vi "CSM - Global Log Event.vi"(6 "timeout in ms (5000ms)":i32=5000, 8 "Error in":errorcluster caption="Error in (no error)") -> (0 "Error out":errorcluster, 3 "CSM Global Log Event":refnum<user-event>)   [LabVIEW 2020, in "Communicable State Machine.lvlib"]
doc: "Obtain CSM Global Log Event Reference.\n\n<b>Inputs:</b>\n - <b>Error in</b>: Error cluster\n\n<b>Outputs:</b>\n - <b>CSM Global Log Event</b>: User event reference for CSM global log.\n - <b>Error out</b>: Error cluster"
uses:
  Communicable State Machine.lvlib
  _CSM_GlobalLog_MSG.ctl
  _CSM_Response Source Message.ctl
  _CSM_GlobalLog_MSG_TYPE.ctl
  GEvt-RequestDef.ctl
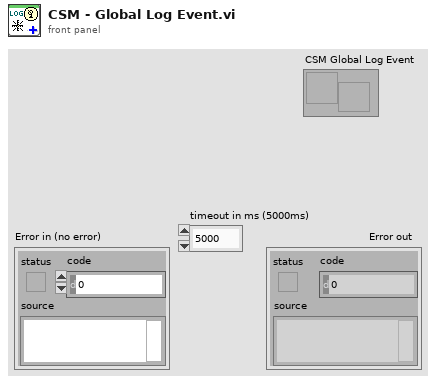
[diagram p1: front panel]
types:
  T1 = typedef "Communicable State Machine.lvlib/GEvt-RequestDef.ctl" = cluster{"Operation":enum16{"Obtain", "Destroy", "Force Destroy"}, "RespQ":refnum<queue>, "CSM Global Log Event":refnum<user-event>}
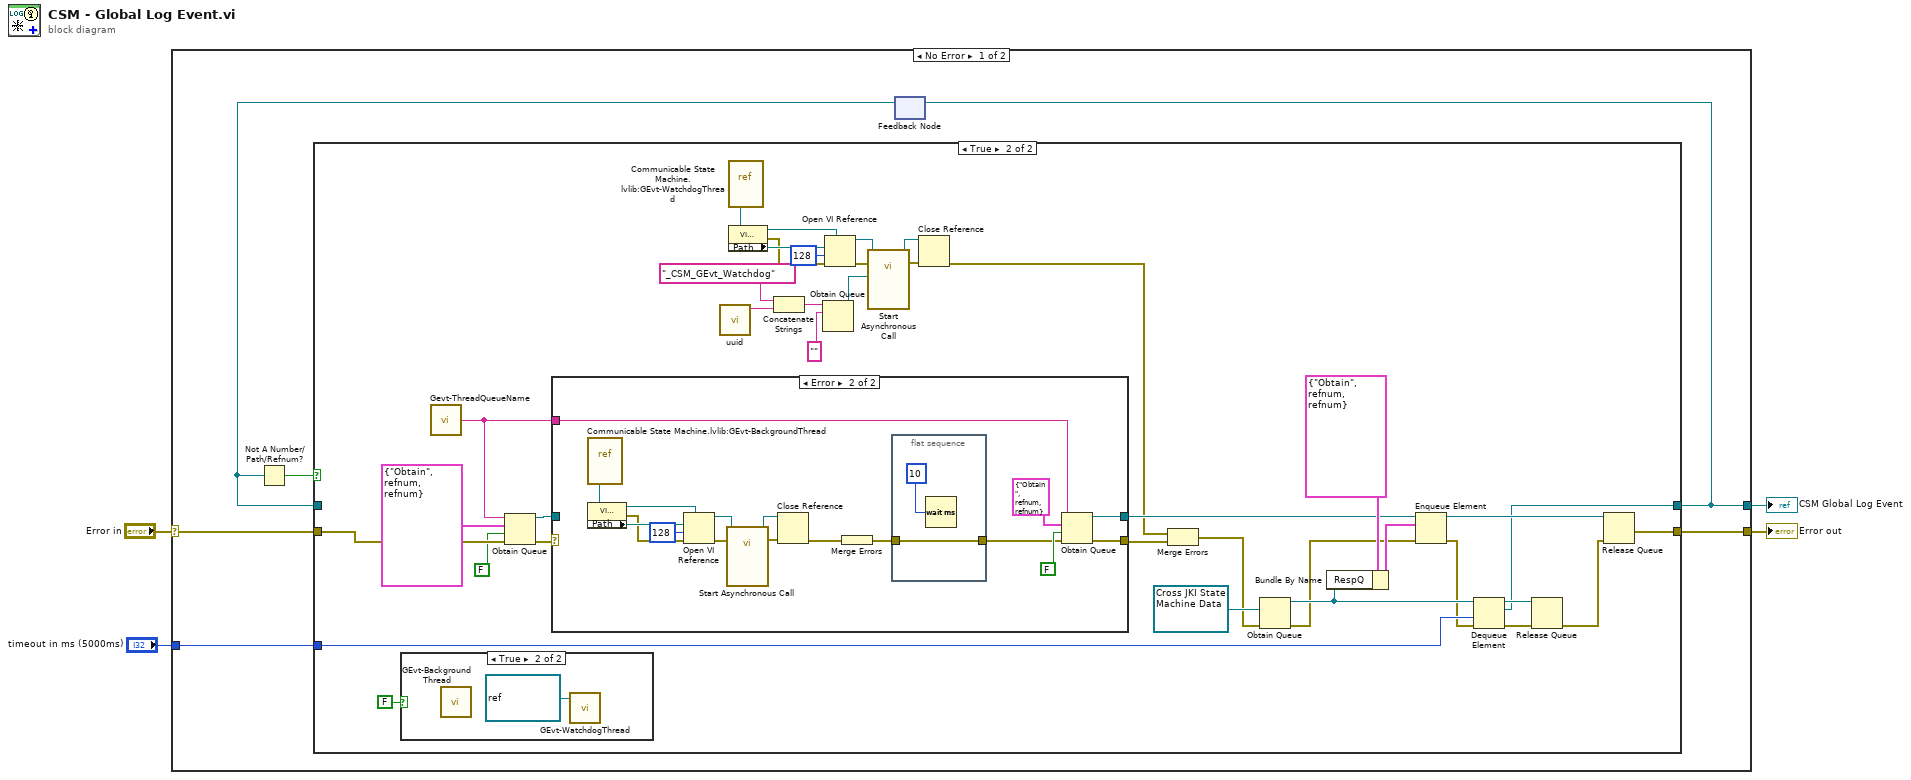
[diagram p0: block diagram]
diagram:
  n1 = case shown="No Error" "Error in" {
    selector: "Error in" -> [w8 w73]
    tunnel: [w10 w73] -> w4
    tunnel: [w7 _] -> w2
    tunnel: "timeout in ms (5000ms)" -> [w9 _]
    frame No Error {
      n2 = feedback #1() -> (w5:refnum<user-event>)  [unwired: 1 in]
      n3 = Not A Number/Path/Refnum?(number/path/refnum=w5) -> (NaN/Path/Refnum?=w6:bool)
      n4 = case shown="True" w6 {
        tunnel: [w11 w50] -> w10
        tunnel: w9 -> [_ w49]
        tunnel: w8 -> [w11 w48]
        tunnel: [w12 w29] -> w7
        tunnel: w5 -> [w12 _]
        frame False {
        }
        frame True {
          n5 = case shown="True" FALSE {
            frame False {
            }
            frame True {
              n6 = call "GEvt-BackgroundThread.vi"() -> ()  [unwired: 12 in]
              n7 = call "GEvt-WatchdogThread.vi"("WatchDogQ"=refnum<queue> refnum) -> ()  [unwired: 11 in]
            }
          }
          n8 = call "Gevt-ThreadQueueName.vi"() -> ("ThreadQueueName"=w31:string)  [unwired: 5 in]
          n9 = Obtain Queue(name (unnamed)=w31, element data type=T1 {"Operation"=enum."Obtain", "RespQ"=refnum, "CSM Global Log Event"=refnum}, create if not found? (T)=FALSE, error in (no error)=w48) -> (queue out=w44:refnum<queue>, error out=w45:errorcluster)  [unwired: 1 in, 1 out]
          n10 = case shown="Error" w45 {
            selector: w45 -> [w53 _]
            tunnel: w44 -> [w52 _]
            tunnel: [w53 w57] -> w38
            tunnel: [w52 w56] -> w39
            tunnel: w31 -> [_ w55]
            frame No Error {
            }
            frame Error {
              n11 = vi-ref "Communicable State Machine.lvlib:GEvt-BackgroundThread.vi"() -> (w69:refnum<vi>)
              n12 = property class="VI (strict)"(reference=w69) -> (reference out=w65:refnum<vi>, error out=w67:errorcluster, "Path"=w68:path)  [unwired: 1 in]
              n13 = Open VI Reference(type specifier VI Refnum (for type only)=w65, vi path=w68, options=128, error in (no error)=w67) -> (vi reference=w66:refnum<vi>, error out=w70:errorcluster)  [unwired: 2 in]
              n14 = call-by-ref "Start Asynchronous Call"(reference=w66, error in=w70) -> (reference out=w63:refnum<vi>, error out=w64:errorcluster)  [unwired: 12 in]
              n15 = Close Reference(reference=w63, error in (no error)=w64) -> (error out=w61:errorcluster)
              n16 = Merge Errors(w61) -> (w54:errorcluster)
              n17 = flat-sequence {
                tunnel: [w71] -> w58
                tunnel: w54 -> [w71]
                frame #0 {
                  n18 = Wait (ms)(milliseconds to wait=u32 10) -> ()  [unwired: 1 out]
                }
              }
              n19 = Obtain Queue(name (unnamed)=w55, element data type=T1 {"Operation"=enum."Obtain", "RespQ"=refnum, "CSM Global Log Event"=refnum}, create if not found? (T)=FALSE, error in (no error)=w58) -> (queue out=w56:refnum<queue>, error out=w57:errorcluster)  [unwired: 1 in, 1 out]
            }
          }
          n20 = call "uuid.vi"() -> ("UUID"=w24:string)  [unwired: 11 in]
          n21 = vi-ref "Communicable State Machine.lvlib:GEvt-WatchdogThread.vi"() -> (w22:refnum<vi>)
          n22 = property class="VI (strict)"(reference=w22) -> (reference out=w18:refnum<vi>, error out=w20:errorcluster, "Path"=w21:path)  [unwired: 1 in]
          n23 = Concatenate Strings("_CSM_GEvt_Watchdog" ("string"), w24) -> (w27:string)
          n24 = Obtain Queue(name (unnamed)=w27, element data type="" ("string")) -> (queue out=w28:refnum<queue>)  [unwired: 3 in, 2 out]
          n25 = Open VI Reference(type specifier VI Refnum (for type only)=w18, vi path=w21, options=128, error in (no error)=w20) -> (vi reference=w19:refnum<vi>, error out=w23:errorcluster)  [unwired: 2 in]
          n26 = call-by-ref "Start Asynchronous Call"(reference=w19, error in=w23, "WatchDogQ"=w28) -> (reference out=w16:refnum<vi>, error out=w17:errorcluster)  [unwired: 11 in]
          n27 = Close Reference(reference=w16, error in (no error)=w17) -> (error out=w13:errorcluster)
          n28 = Merge Errors(w13, w38) -> (w14:errorcluster)
          n29 = Obtain Queue(element data type=refnum<user-event> refnum ("CSM Global Log Event"), error in (no error)=w14) -> (queue out=w40:refnum<queue>, error out=w37:errorcluster)  [unwired: 3 in, 1 out]
          n30 = Bundle By Name(cluster=T1 {"Operation"=enum."Obtain", "RespQ"=refnum, "CSM Global Log Event"=refnum} ("element"), "RespQ"=w40) -> (w42:T1)
          n31 = Enqueue Element(queue=w39, element=w42, error in (no error)=w37) -> (queue out=w33:refnum<queue>, error out=w36:errorcluster)  [unwired: 1 in, 1 out]
          n32 = Dequeue Element(queue=w40, timeout in ms (-1)=w49, error in (no error)=w36) -> (queue out=w34:refnum<queue>, element=w29:refnum<user-event>, error out=w35:errorcluster)  [unwired: 1 out]
          n33 = Release Queue(queue=w34, error in (no error)=w35) -> (error out=w32:errorcluster)  [unwired: 1 in, 2 out]
          n34 = Release Queue(queue=w33, error in (no error)=w32) -> (error out=w50:errorcluster)  [unwired: 1 in, 2 out]
        }
      }
      n35 = feedback-in #1(w7) -> ()
    }
    frame Error {
    }
  }
  "Error out" <- w4
  "CSM Global Log Event" <- w2
